vi "DLL Get Status.vi"(8 "error in (no error)":errorcluster, 11 "Phasor Data Concentrator in":refnum<class "Phasor Data Concentrator.lvclass">) -> (0 "error out":errorcluster, 1 "Configuration File Received":bool, 2 "Timeout":bool, 3 "Phasor Data Concentrator out":refnum<class "Phasor Data Concentrator.lvclass">, 4 "Configuration Read OK":bool, 5 "PDC Connected":bool, 7 "Data Rate":sgl)   [LabVIEW 2013, in "PMU Recorder Light.lvlib" / "Phasor Data Concentrator.lvclass"]
doc: "Gets the status indicators from the DLL"
uses:
  Phasor Data Concentrator.lvclass
  Statnett C37.118 DLL/Statnett C37.118 DLL.lvclass
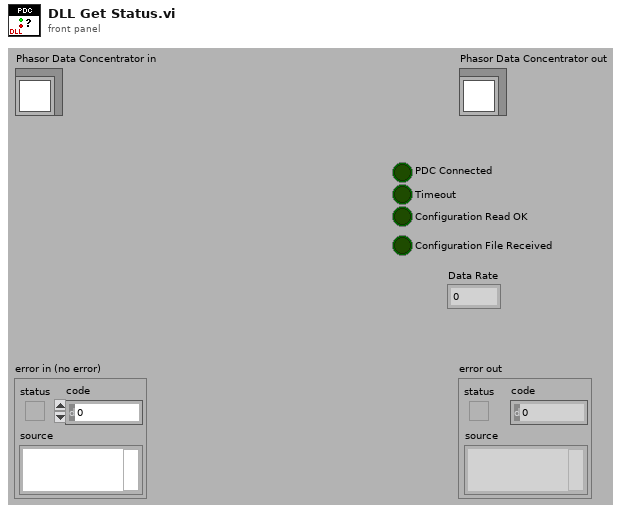
[diagram p1: front panel]
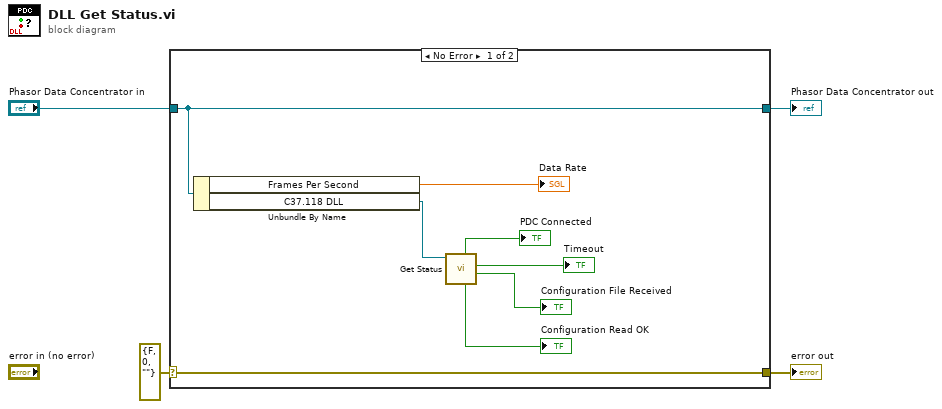
[diagram p0: block diagram]
diagram:
  n1 = case shown="No Error" errorcluster {"status"=FALSE, "code"=0, "source"=""} ("error IO") {
    selector: errorcluster {"status"=FALSE, "code"=0, "source"=""} ("error IO") -> [w12 w14]
    tunnel: [w12 w14] -> w4
    tunnel: [w11 w13] -> w2
    tunnel: "Phasor Data Concentrator in" -> [w11 w13]
    frame No Error {
      n2 = Unbundle By Name(w11) -> ("Frames Per Second"=→"Data Rate":sgl, "C37.118 DLL"=w9:refnum<class "Statnett C37.118 DLL.lvclass">)
      n3 = call "Get Status.vi"("Statnett C37.118 DLL in"=w9) -> ("Configuration File Received"=→"Configuration File Received":bool, "Timeout"=→"Timeout":bool, "Configuration Read OK"=→"Configuration Read OK":bool, "PDC Connected"=→"PDC Connected":bool)  [unwired: 5 in, 2 out]
    }
    frame Error {
    }
  }
  "error out" <- w4
  "Phasor Data Concentrator out" <- w2
